vi "HostMain.vi"() -> ()   [LabVIEW 2017]
doc: "Main VI to be run from host computer. Can be started before or after the cRIO VI, RTMain.vi"
uses:
  RTControl/StateList.ctl
  HostDataGLOBAL.vi
  SystemsCheckPressureLimitGLOBAL.vi
  HostCurrentTimeGLOBAL.vi
  <vilib>/Utility/file.llb/Write Delimited Spreadsheet (string).vi
  <vilib>/Utility/file.llb/Write Delimited Spreadsheet (DBL).vi
panel:
  in  "Vent Tubing":bool
  out "Distance":dbl(slide) scale=0.0..1609.0
  in  "Skip System Check":bool
  in  "Stop System Check":bool
  in  "Enable Pod Power":string
  in  "Vent Tanks":bool
  out "Acceleration Graph":cluster{dbl[], dbl[]}(graph)
  out "Speed Graph":cluster{dbl[], dbl[]}(graph)
  out "Emergency Source":string
  out "Health Check 2":T1(array[cluster])=[{"String"="Distance (m)", "Numeric"=0.0, "Boolean"=FALSE}, {"String"="Piezo (V)", "Numeric"=0.0, "Boolean"=FALSE}, {"String"="Battery Voltage (V)", "Numeric"=0.0, "Boolean"=FALSE}, {"String"="Battery Current (I)", "Numeric"=0.0, "Boolean"=FALSE}, {"String"="Battery Power (W)", "Numeric"=0.0, "Boolean"=FALSE}, {"String"="Battery Temperature (C)", "Numeric"=0.0, "Boolean"=FALSE}, {"String"="cRIO Temperature (C)", "Numeric"=0.0, "Boolean"=FALSE}, {"String"="Right Big Tank Temperature (C)", "Numeric"=0.0, "Boolean"=FALSE}, {"String"="Left Big Tank Temperature (C)", "Numeric"=0.0, "Boolean"=FALSE}, {"String"="Baby Tank Temperature (C)", "Numeric"=0.0, "Boolean"=FALSE}, {"String"="Right Manifold Temperature (C)", "Numeric"=0.0, "Boolean"=FALSE}, {"String"="Left Manifold Temperature (C)", "Numeric"=0.0, "Boolean"=FALSE}, {"String"="IMU Acceleration", "Numeric"=0.0, "Boolean"=FALSE}, {"String"="IMU Pressure", "Numeric"=0.0, "Boolean"=FALSE}, {"String"="IMU Temperature", "Numeric"=0.0, "Boolean"=FALSE}]
  out "End Coast Time":dbl=-0.01
  out "End Push Time":dbl=-0.01
  out "Start Push Time":dbl=-0.01
  out "Current Time":dbl=-0.01
  in  "Force Idle":bool
  in  "Testing Mode?":bool
  out "Health Check":T1(array[cluster])=[{"String"="Suspension Pressure (PSI)", "Numeric"=0.0, "Boolean"=FALSE}, {"String"="MagBrake Pressure (PSI)", "Numeric"=0.0, "Boolean"=FALSE}, {"String"="Small Tank (PSI)", "Numeric"=0.0, "Boolean"=FALSE}, {"String"="Big Tank Right (PSI)", "Numeric"=0.0, "Boolean"=FALSE}, {"String"="Big Tank Left (PSI)", "Numeric"=0.0, "Boolean"=FALSE}, {"String"="FL Hall Effect (V)", "Numeric"=0.0, "Boolean"=FALSE}, {"String"="FR Hall Effect (V)", "Numeric"=0.0, "Boolean"=FALSE}, {"String"="BR Hall Effect (V)", "Numeric"=0.0, "Boolean"=FALSE}, {"String"="BL Hall Effect (V)", "Numeric"=0.0, "Boolean"=FALSE}, {"String"="FR Linear Pot (V)", "Numeric"=0.0, "Boolean"=FALSE}, {"String"="FL Linear Pot (V)", "Numeric"=0.0, "Boolean"=FALSE}, {"String"="BR Linear Pot (V)", "Numeric"=0.0, "Boolean"=FALSE}, {"String"="BL Linear Pot (V)", "Numeric"=0.0, "Boolean"=FALSE}, {"String"="Speed (m/s)", "Numeric"=0.0, "Boolean"=FALSE}]
  out "UDP String":string
  in  "Emergency":bool
  in  "Clear Error":bool
  in  "Abort":bool
  out "CurrentState":T2
  in  "Idle to Ready":bool
  in  "Power On":bool
  in  "Stop Host":bool
  in  "Stop cRIO":bool
  out "Solenoid Tabs":enum32{"System Check", "State Machine"}(tab)
  in  "All Toggle On":bool
  in  "All Toggle Off":bool
  in  "Manual Control":bool
  in  "NC09":bool
  in  "NO01":bool
  in  "NC08":bool
  in  "NC05":bool
  in  "NC06":bool
  in  "NC07":bool
  in  "NC03":bool
  in  "NC04":bool
  in  "NC02":bool
  in  "NC10":bool
  in  "NO02":bool
  in  "NC01":bool
  in  "Mag Brake Toggle":bool
  in  "Suspension Toggle":bool
  in  "Levitation Toggle":bool
  out "Left Solenoids":cluster{"String":string, "Boolean":bool}[](array[cluster])=[{"String"="NC03 FLSki", "Boolean"=FALSE}, {"String"="NC04 BLSki", "Boolean"=FALSE}, {"String"="NC02 BLSki", "Boolean"=FALSE}, {"String"="NC10 MagBr In", "Boolean"=FALSE}, {"String"="NO02 MagBr Out", "Boolean"=FALSE}, {"String"="NC01 FLSki", "Boolean"=FALSE}, {"String"="Pod Power", "Boolean"=FALSE}]
  out "Right Solenoids":cluster{"String":string, "Boolean":bool}[](array[cluster])=[{"String"="NC09 Susp In", "Boolean"=FALSE}, {"String"="NO01 Susp Out", "Boolean"=FALSE}, {"String"="NC08 BRSki", "Boolean"=FALSE}, {"String"="NC05 FRSki", "Boolean"=FALSE}, {"String"="NC06 BRSki", "Boolean"=FALSE}, {"String"="NC07 FRSki", "Boolean"=FALSE}, {"String"="NO03 All Out", "Boolean"=FALSE}, {"String"="Safety Panel", "Boolean"=FALSE}]
  # "IN"
  # "IN"
  # "MAG"
  # "SUSP"
  # "OUT"
  # "OUT"
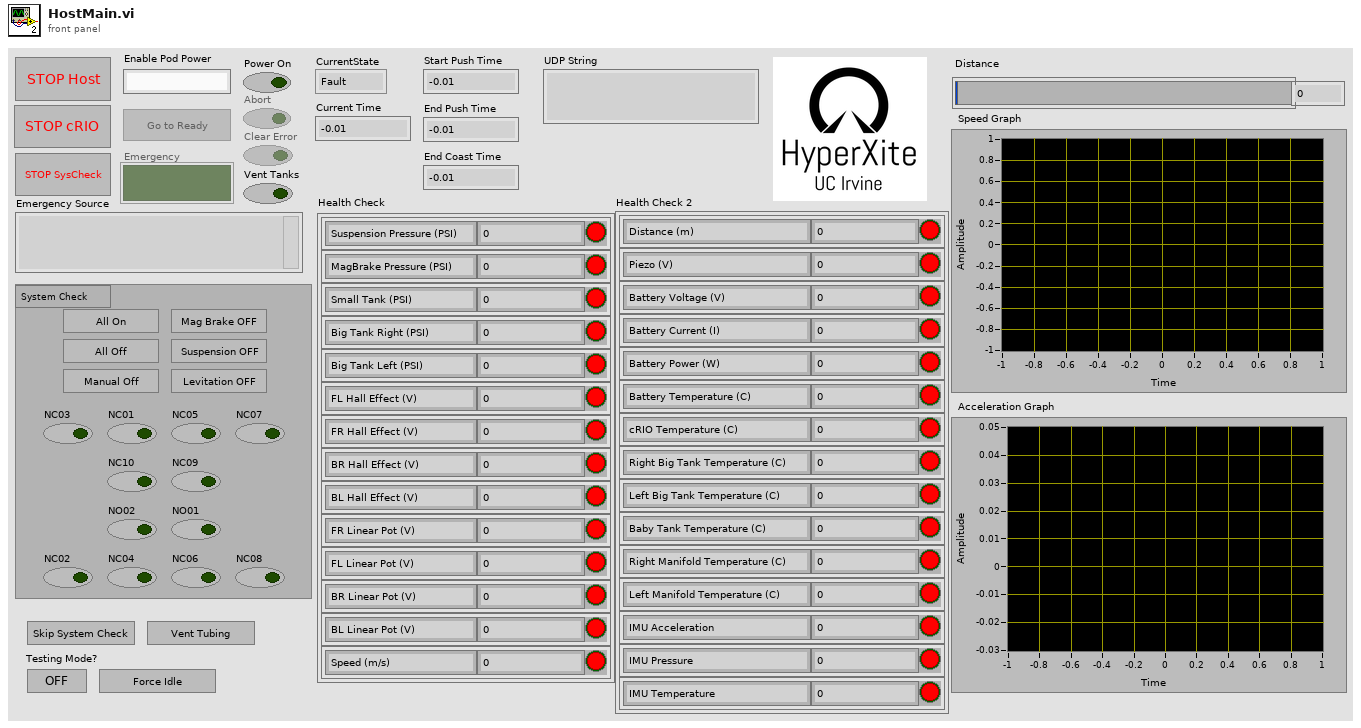
[diagram p1: front panel]
types:
  T1 = cluster{"String":string, "Numeric":dbl, "Boolean":bool}[]
  T2 = typedef "StateList.ctl" = enum16{"Fault", "Idle", "Ready", "Pushing", "Coast", "Braking"}
  T3 = enum8{"Enabled", "Disabled", "Disabled and Grayed Out"}
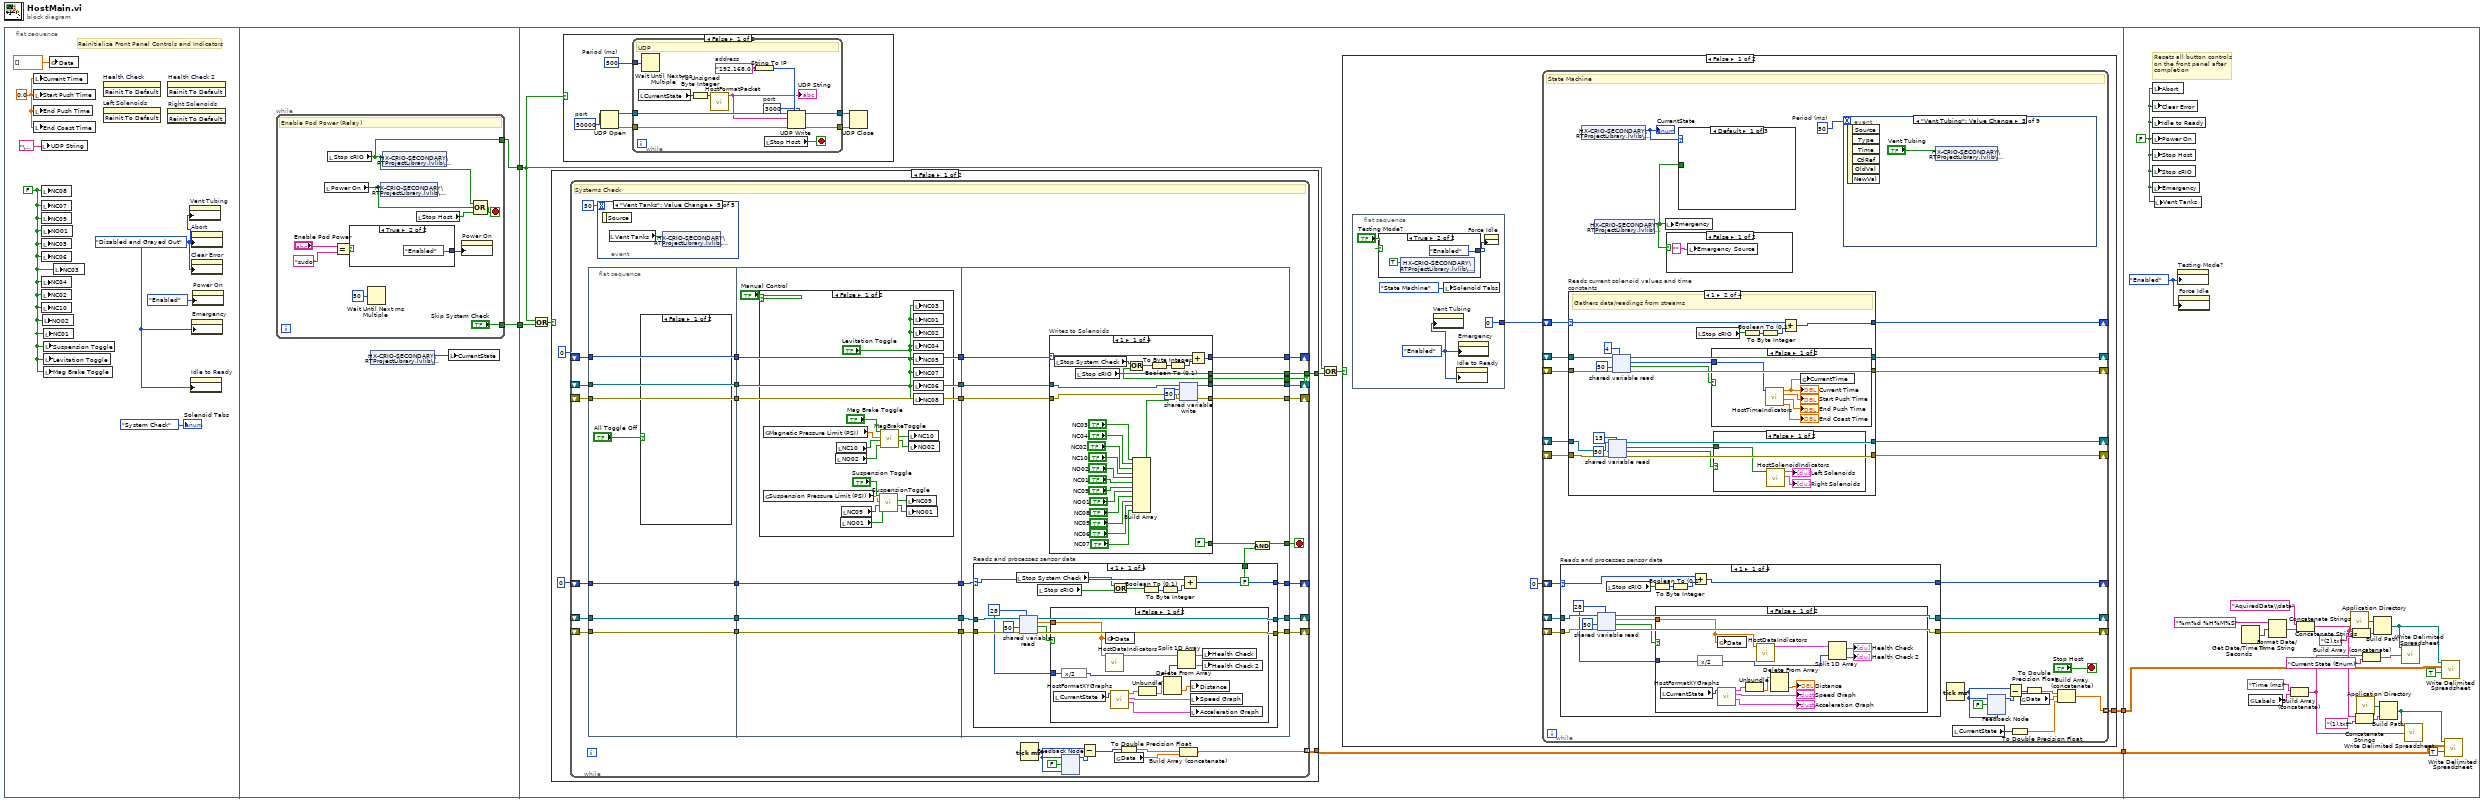
[diagram p0: block diagram]
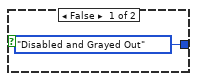
[diagram p2: hidden frame]
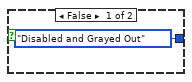
[diagram p4: hidden frame]
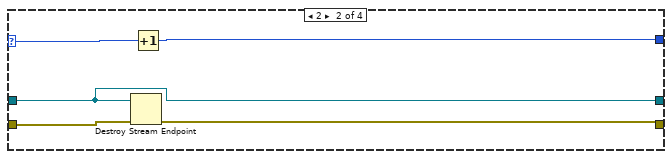
[diagram p6: hidden frame]
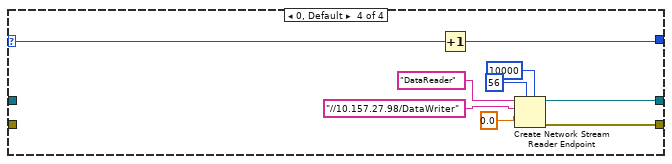
[diagram p8: hidden frame]
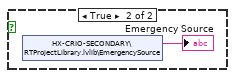
[diagram p9: hidden frame]
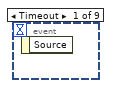
[diagram p10: hidden frame]
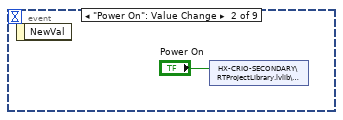
[diagram p11: hidden frame]
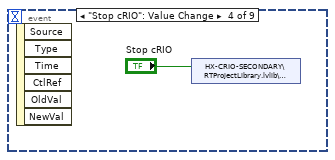
[diagram p12: hidden frame]
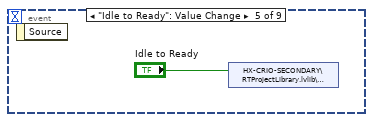
[diagram p13: hidden frame]
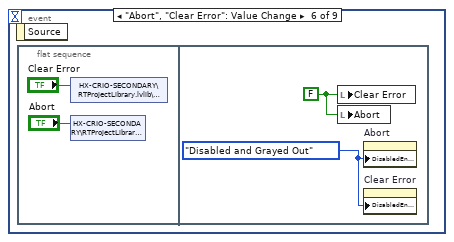
[diagram p14: hidden frame]
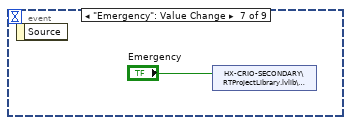
[diagram p15: hidden frame]
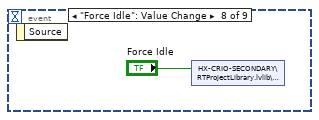
[diagram p16: hidden frame]
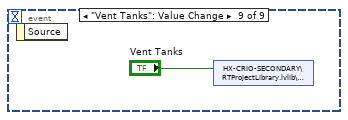
[diagram p17: hidden frame]
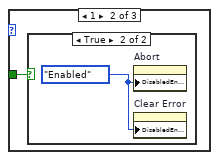
[diagram p18: hidden frame]
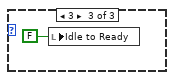
[diagram p20: hidden frame]
diagram:
  n1 = flat-sequence {
    tunnel: [w14] -> w4
    tunnel: [w13] -> w3
    tunnel: w4 -> [w32]
    tunnel: w3 -> [w27]
    tunnel: [w29] -> w2
    tunnel: [w28] -> w1
    tunnel: w2 -> [w412]
    tunnel: w1 -> [w411]
    frame #0 {
      w5 = T3."Disabled and Grayed Out" ("Disabled")
      w6 = FALSE
      w10 = 0.0 ("Speed (m/s)")
      # "Reinitialize Front Panel Controls and Indicators"
      n2 = local write "Current Time"(w10) -> ()
      n3 = local write "Start Push Time"(w10) -> ()
      n4 = local write "End Push Time"(w10) -> ()
      n5 = local write "End Coast Time"(w10) -> ()
      n6 = local write "UDP String"("\u0000\u0000\u0000\u0000\u0000\u0000\u0000\u0000\u0000\u0000\u0000\u0000\u0000\u0000\u0000\u0000\u0000\u0000\u0000\u0000\u0000\u0000\u0000\u0000\u0000\u0000\u0000\u0000\u0000\u0000\u0000\u0000\u0000\u0000" ("UDP String")) -> ()
      n7 = local write "NC08"(w6) -> ()
      n8 = local write "NC07"(w6) -> ()
      n9 = local write "NC09"(w6) -> ()
      n10 = local write "NO01"(w6) -> ()
      n11 = local write "NC05"(w6) -> ()
      n12 = local write "NC06"(w6) -> ()
      n13 = local write "NC04"(w6) -> ()
      n14 = local write "NC02"(w6) -> ()
      n15 = local write "NC10"(w6) -> ()
      n16 = local write "NO02"(w6) -> ()
      n17 = local write "NC01"(w6) -> ()
      n18 = local write "Suspension Toggle"(w6) -> ()
      n19 = local write "Levitation Toggle"(w6) -> ()
      n20 = local write "Mag Brake Toggle"(w6) -> ()
      n21 = global write "HostDataGLOBAL.vi" "Data"(dbl[] [] ("Data")) -> ()
      n22 = local write "NC03"(w6) -> ()
      n23 = invoke on="Health Check" class="Arr (strict)" method="Reinit To Default"() -> ()  [unwired: 3 in, 3 out]
      n24 = invoke on="Left Solenoids" class="Arr (strict)" method="Reinit To Default"() -> ()  [unwired: 3 in, 3 out]
      n25 = invoke on="Health Check 2" class="Arr (strict)" method="Reinit To Default"() -> ()  [unwired: 3 in, 3 out]
      n26 = invoke on="Right Solenoids" class="Arr (strict)" method="Reinit To Default"() -> ()  [unwired: 3 in, 3 out]
      n27 = property on="Vent Tubing" class="Bool (strict)"("DisabledEnum"=w5) -> ()  [unwired: 2 in, 2 out]
      n28 = property on="Idle to Ready" class="Bool (strict)"("DisabledEnum"=w5) -> ()  [unwired: 2 in, 2 out]
      n29 = property on="Abort" class="Bool (strict)"("DisabledEnum"=w5) -> ()  [unwired: 2 in, 2 out]
      n30 = property on="Clear Error" class="Bool (strict)"("DisabledEnum"=w5) -> ()  [unwired: 2 in, 2 out]
      n31 = property on="Emergency" class="Bool (strict)"("DisabledEnum"=w5) -> ()  [unwired: 2 in, 2 out]
      n32 = property on="Power On" class="Bool (strict)"("DisabledEnum"=T3."Enabled" ("Disabled")) -> ()  [unwired: 2 in, 2 out]
      "Solenoid Tabs" <- enum32{"System Check", "State Machine"}."System Check" ("Solenoid Tabs")
    }
    frame #1 {
      n33 = while {
        tunnel: ["Skip System Check"] -> w14
        tunnel: [w15] -> w13
        stop <- w23 stop-if-true
        # "Enable Pod Power (Relay)"
        n34 = local read "Power On"() -> (w16:bool)
        n35 = local read "Stop cRIO"() -> (w15:bool)
        n36 = Equal?(x="Enable Pod Power", y="sudo") -> (x = y?=w19:bool)
        n37 = case shown="True" w19 {
          tunnel: [T3."Disabled and Grayed Out" ("Disabled") T3."Enabled" ("Disabled")] -> w18
          frame False {
          }
          frame True {
          }
        }
        n38 = Wait Until Next ms Multiple(millisecond multiple=u32 50) -> ()  [unwired: 1 out]
        n39 = shared-variable "HX-CRIO-SECONDARY\\RTProjectLibrary.lvlib\\PodPower"(w16) -> ()  [unwired: 1 in, 1 out]
        n40 = shared-variable "HX-CRIO-SECONDARY\\RTProjectLibrary.lvlib\\StopControl"(w15) -> ()  [unwired: 1 in, 1 out]
        n41 = local read "Stop Host"() -> (w24:bool)
        n42 = property on="Power On" class="Bool (strict)"("DisabledEnum"=w18) -> ()  [unwired: 2 in, 2 out]
        n43 = Compound Arithmetic op=OR(w15, w16, w24) -> (w23:bool)
      }
      n44 = shared-variable "HX-CRIO-SECONDARY\\RTProjectLibrary.lvlib\\CurrentState"() -> (w12:u8)  [unwired: 1 in, 1 out]
      n45 = local write "CurrentState"(w12) -> ()
    }
    frame #2 {
      n46 = Or(x=w27, y=w32) -> (x .or. y?=w33:bool)
      n47 = case shown="False" w33 {
        selector: w33 -> [_ w399]
        tunnel: [w211 FALSE ("Stop cRIO")] -> w31
        tunnel: [w210 dbl[][] [] ("Data")] -> w28
        frame False {
          n48 = while {
            shift-right: [w246] -> _
            shift-left: i8 0 -> [w247]
            shift-right: [w245] -> _
            shift-left: _ -> [w243]
            shift-right: [w244] -> _
            shift-left: _ -> [w242]
            tunnel: [w233] -> w211 if=w232
            shift-right: [w228] -> _
            shift-left: i8 0 -> [w229]
            shift-right: [w221] -> _
            shift-left: _ -> [w225]
            shift-right: [w220] -> _
            shift-left: _ -> [w222]
            tunnel: [w218] -> w210 mode=indexing
            stop <- w241 stop-if-true
            # "Systems Check"
            n49 = flat-sequence {
              tunnel: w242 -> [w256]
              tunnel: w243 -> [w257]
              tunnel: w247 -> [w258]
              tunnel: [w258] -> w237
              tunnel: [w257] -> w236
              tunnel: [w256] -> w235
              tunnel: [w254] -> w230
              tunnel: w229 -> [w254]
              tunnel: [w253] -> w226
              tunnel: w225 -> [w253]
              tunnel: [w252] -> w223
              tunnel: w222 -> [w252]
              tunnel: [w267] -> w240
              tunnel: [w266] -> w239
              tunnel: [w265] -> w238
              tunnel: w237 -> [w267]
              tunnel: w236 -> [w266]
              tunnel: w235 -> [w265]
              tunnel: [w263] -> w231
              tunnel: w230 -> [w263]
              tunnel: [w262] -> w227
              tunnel: w226 -> [w262]
              tunnel: [w261] -> w224
              tunnel: w223 -> [w261]
              tunnel: [w298] -> w246
              tunnel: [w297] -> w245
              tunnel: [w296] -> w244
              tunnel: [w284] -> w241
              tunnel: w240 -> [w299]
              tunnel: w239 -> [w295]
              tunnel: w238 -> [w294]
              tunnel: [w292] -> w233
              tunnel: [w291] -> w232
              tunnel: w231 -> [w290]
              tunnel: [w289] -> w228
              tunnel: w227 -> [w288]
              tunnel: w224 -> [w287]
              tunnel: [w286] -> w221
              tunnel: [w285] -> w220
              frame #0 {
                n50 = case shown="False" "All Toggle Off" {
                  selector: "All Toggle Off" -> [_ w260]
                  frame False {
                  }
                  frame True {
                    n51 = Not(x=w260) -> (.not. x?=w259:bool)
                    n52 = local write "Suspension Toggle"(w259) -> ()
                    n53 = local write "Mag Brake Toggle"(w259) -> ()
                    n54 = local write "Levitation Toggle"(w259) -> ()
                    n55 = local write "NO01"(w259) -> ()
                    n56 = local write "NO02"(w259) -> ()
                    n57 = local write "NC08"(w259) -> ()
                    n58 = local write "NC07"(w259) -> ()
                    n59 = local write "NC09"(w259) -> ()
                    n60 = local write "NC05"(w259) -> ()
                    n61 = local write "NC06"(w259) -> ()
                    n62 = local write "NC03"(w259) -> ()
                    n63 = local write "NC04"(w259) -> ()
                    n64 = local write "NC02"(w259) -> ()
                    n65 = local write "NC10"(w259) -> ()
                    n66 = local write "NC01"(w259) -> ()
                  }
                }
              }
              frame #1 {
                n67 = case shown="False" "Manual Control" {
                  frame False {
                    n68 = global read "SystemsCheckPressureLimitGLOBAL.vi" "Magnetic Pressure Limit (PSI)"() -> (w269:dbl)
                    n69 = global read "SystemsCheckPressureLimitGLOBAL.vi" "Suspension Pressure Limit (PSI)"() -> (w268:dbl)
                    n70 = local read "NO02"() -> (w278:bool)
                    n71 = local read "NC10"() -> (w277:bool)
                    n72 = local read "NO01"() -> (w280:bool)
                    n73 = local read "NC09"() -> (w279:bool)
                    n74 = call "SuspensionToggle.vi"("Susp Out"=w280, "SuspIn"=w279, "Suspension Pressure Limit (PSI)"=w268, "SuspensionOn?"="Suspension Toggle") -> ("SuspOut"=w275:bool, "SuspIn"=w276:bool)  [unwired: 5 in, 1 out]
                    n75 = call "MagBrakeToggle.vi"("MagBrake Out"=w278, "MagBrake In"=w277, "MagPressureLimit (PSI)"=w269, "MagBrakeOn?"="Mag Brake Toggle") -> ("MagBrake OUTPUT"=w274:bool, "MagBrake In"=w273:bool)  [unwired: 5 in, 1 out]
                    n76 = local write "NC09"(w276) -> ()
                    n77 = local write "NO01"(w275) -> ()
                    n78 = local write "NC10"(w273) -> ()
                    n79 = local write "NO02"(w274) -> ()
                    n80 = local write "NC03"("Levitation Toggle") -> ()
                    n81 = local write "NC01"("Levitation Toggle") -> ()
                    n82 = local write "NC02"("Levitation Toggle") -> ()
                    n83 = local write "NC04"("Levitation Toggle") -> ()
                    n84 = local write "NC05"("Levitation Toggle") -> ()
                    n85 = local write "NC07"("Levitation Toggle") -> ()
                    n86 = local write "NC06"("Levitation Toggle") -> ()
                    n87 = local write "NC08"("Levitation Toggle") -> ()
                  }
                  frame True {
                    n88 = case shown="True" "All Toggle On" {
                      selector: "All Toggle On" -> [_ w282]
                      frame False {
                      }
                      frame True {
                        n89 = local write "NC08"(w282) -> ()
                        n90 = local write "NC07"(w282) -> ()
                        n91 = local write "NC09"(w282) -> ()
                        n92 = local write "NO01"(w282) -> ()
                        n93 = local write "NC05"(w282) -> ()
                        n94 = local write "NC06"(w282) -> ()
                        n95 = local write "NC03"(w282) -> ()
                        n96 = local write "NC04"(w282) -> ()
                        n97 = local write "NC02"(w282) -> ()
                        n98 = local write "NC10"(w282) -> ()
                        n99 = local write "NO02"(w282) -> ()
                        n100 = local write "NC01"(w282) -> ()
                      }
                    }
                  }
                }
              }
              frame #2 {
                n101 = case "Reads and processes sensor data" shown="1" w290 {
                  selector: w290 -> [w310 w333 w337 w343]
                  tunnel: [w311 w332 w337 w342] -> w289
                  tunnel: [w309 w329 w336 w341] -> w286
                  tunnel: [w308 w330 w335 w340] -> w285
                  tunnel: w288 -> [w312 w329 w336 _]
                  tunnel: w287 -> [w313 w331 w335 _]
                  tunnel: [FALSE FALSE TRUE FALSE] -> w283
                  frame 1 {
                    w303 = 28 ("# elements")
                    n102 = local read "Stop System Check"() -> (w304:bool)
                    n103 = shared-variable-read(w312, w313, 50 ("timeout ms (-1)"), w303) -> (w309:refnum<k21>, w308:errorcluster, w300:bool, w302:dbl[])
                    n104 = local read "Stop cRIO"() -> (w306:bool)
                    n105 = case shown="False" w300 {
                      tunnel: w303 -> [w323 _]
                      tunnel: w302 -> [w321 _]
                      frame False {
                        n106 = local read "CurrentState"() -> (w325:T2)
                        n107 = expression code="x/2"(w323) -> (w324:i32)
                        n108 = global write "HostDataGLOBAL.vi" "Data"(w321) -> ()
                        n109 = call "HostDataIndicators.vi"("Array"=w321) -> ("Health Check"=w322:T1)  [unwired: 10 in]
                        n110 = call "HostFormatXYGraphs.vi"("CurrentState"=w325) -> ("Acceleration Graph"=w318:cluster{dbl[], dbl[]}, "Speed Graph"=w317:cluster{dbl[], dbl[]}, "Distance Graph"=w326:cluster{dbl[], dbl[]})  [unwired: 8 in]
                        n111 = Unbundle(w326) -> (w327:dbl[])  [unwired: 1 out]
                        n112 = Delete From Array(array=w327) -> (deleted portion=w316:dbl)  [unwired: 2 in, 1 out]
                        n113 = Split 1D Array(array=w322, index=w324) -> (first subarray=w320:T1, second subarray=w319:T1)
                        n114 = local write "Distance"(w316) -> ()
                        n115 = local write "Speed Graph"(w317) -> ()
                        n116 = local write "Acceleration Graph"(w318) -> ()
                        n117 = local write "Health Check"(w320) -> ()
                        n118 = local write "Health Check 2"(w319) -> ()
                      }
                      frame True {
                      }
                    }
                    n119 = Or(x=w304, y=w306) -> (x .or. y?=w305:bool)
                    n120 = Boolean To (0,1)(Boolean=w305) -> (0, 1=w314:i16)
                    n121 = To Byte Integer(number=w314) -> (8bit integer=w315:i8)
                    n122 = Add(x=w310, y=w315) -> (x+y=w311:i8)
                  }
                  frame 2 {
                    n123 = Destroy Stream Endpoint(8:w331, 11:w329) -> (0:w330:errorcluster)
                    n124 = Increment(x=w333) -> (x+1=w332:i8)
                  }
                  frame 3 {
                  }
                  frame 0, Default {
                    n125 = Increment(x=w343) -> (x+1=w342:i8)
                    n126 = Create Network Stream Reader Endpoint(5:10000 ("timeout in ms (-1)"), 7:56 ("reader buffer size"), 9:0.0, 10:"//10.157.27.98/DataWriter" ("writer url"), 11:"DataReader" ("reader name")) -> (0:w340:errorcluster, 3:w341:refnum<k21>)  [unwired: 2 in]
                  }
                }
                n127 = case "Writes to Solenoids" shown="1" w299 {
                  selector: w299 -> [w371 w377 w381 w392]
                  tunnel: [w368 w374 w381 w391] -> w298
                  tunnel: [w369 w378 w383 w390] -> w297
                  tunnel: [w370 w379 w384 w389] -> w296
                  tunnel: w295 -> [w349 w378 w383 _]
                  tunnel: w294 -> [w350 w380 w384 _]
                  tunnel: [FALSE FALSE TRUE FALSE] -> w293
                  tunnel: [w353 w375 w382 FALSE ("Stop cRIO")] -> w292
                  tunnel: [w353 w375 w382 TRUE ("Stop cRIO")] -> w291
                  frame 1 {
                    n128 = local read "Stop System Check"() -> (w351:bool)
                    n129 = local read "Stop cRIO"() -> (w353:bool)
                    n130 = Or(x=w351, y=w353) -> (x .or. y?=w352:bool)
                    n131 = Build Array("NC03", "NC04", "NC02", "NC10", "NO02", "NC01", "NC09", "NO01", "NC08", "NC05", "NC06", "NC07") -> (w355:bool[])
                    n132 = Boolean To (0,1)(Boolean=w352) -> (0, 1=w372:i16)
                    n133 = To Byte Integer(number=w372) -> (8bit integer=w373:i8)
                    n134 = shared-variable-write(w349, w350, w355, 50 ("timeout ms (-1)")) -> (w369:refnum<k21>, w370:errorcluster)  [unwired: 1 out]
                    n135 = Add(x=w371, y=w373) -> (x+y=w368:i8)
                  }
                  frame 2 {
                    w375 = FALSE ("Stop cRIO")
                    n136 = Destroy Stream Endpoint(8:w380, 11:w378) -> (0:w379:errorcluster)
                    n137 = Increment(x=w377) -> (x+1=w374:i8)
                  }
                  frame 3 {
                    w382 = FALSE ("Stop cRIO")
                  }
                  frame 0, Default {
                    n138 = Increment(x=w392) -> (x+1=w391:i8)
                    n139 = Create Network Stream Writer Endpoint(7:24 ("reader buffer size"), 9:FALSE, 10:"//10.157.27.98/ManuelWriter" ("writer url"), 11:"ManuelReader" ("reader name")) -> (0:w389:errorcluster, 3:w390:refnum<k21>)  [unwired: 3 in]
                  }
                }
                n140 = And(x=w293, y=w283) -> (x .and. y?=w284:bool)
              }
            }
            n141 = event shown="[4] \"Vent Tanks\": Value Change" {
              selector: _ -> [_ _ _ _ _]
              dyn-events: _ -> [_ _ _ _ _]
              timeout: 50 -> [_ _ _ _ _]
              event Timeout {
                n142 = event-data() -> ()  [unwired: 1 in, 1 out]
              }
              event "Stop System Check": Value Change {
                n143 = event-data() -> ()  [unwired: 1 in, 1 out]
                n144 = shared-variable "HX-CRIO-SECONDARY\\RTProjectLibrary.lvlib\\StopSystemCheck"("Stop System Check") -> ()  [unwired: 1 in, 1 out]
              }
              event "Power On": Value Change {
                n145 = event-data() -> ()  [unwired: 1 in, 1 out]
                n146 = local read "Power On"() -> (w249:bool)
                n147 = shared-variable "HX-CRIO-SECONDARY\\RTProjectLibrary.lvlib\\PodPower"(w249) -> ()  [unwired: 1 in, 1 out]
              }
              event "Stop cRIO": Value Change {
                n148 = event-data() -> ()  [unwired: 1 in, 1 out]
                n149 = local read "Stop cRIO"() -> (w250:bool)
                n150 = shared-variable "HX-CRIO-SECONDARY\\RTProjectLibrary.lvlib\\StopControl"(w250) -> ()  [unwired: 1 in, 1 out]
              }
              event "Vent Tanks": Value Change {
                n151 = event-data() -> ()  [unwired: 1 in, 1 out]
                n152 = local read "Vent Tanks"() -> (w251:bool)
                n153 = shared-variable "HX-CRIO-SECONDARY\\RTProjectLibrary.lvlib\\VentTanks"(w251) -> ()  [unwired: 1 in, 1 out]
              }
            }
            n154 = Tick Count (ms)() -> (millisecond timer value=w214:u32)
            n155 = feedback-in #1(w214, FALSE) -> ()
            n156 = feedback #1(w214) -> (w217:u32)
            n157 = Subtract(x=w214, y=w217) -> (x-y=w216:u32)
            n158 = global read "HostDataGLOBAL.vi" "Data"() -> (w219:dbl[])
            n159 = To Double Precision Float(number=w216) -> (double precision float=w215:dbl)
            n160 = Build Array (concatenate)(w215, w219) -> (w218:dbl[])
          }
        }
        frame True {
          n161 = shared-variable "HX-CRIO-SECONDARY\\RTProjectLibrary.lvlib\\StopSystemCheck"(w399) -> ()  [unwired: 1 in, 1 out]
        }
      }
      n162 = case shown="False" w27 {
        frame False {
          w34 = u32 500  # Period (ms)
          w35 = u16 50000  # port
          n163 = UDP Open(11:w35) -> (port=w36:refnum<k16>, 0:w39:errorcluster)  [unwired: 4 in, 1 out]
          n164 = while {
            tunnel: w39 -> [w50]
            tunnel: [w49] -> w38
            tunnel: [w48] -> w37
            tunnel: w36 -> [w47]
            tunnel: w34 -> [w40]
            stop <- w51 stop-if-true
            w44 = u16 3000  # port
            w45 = "192.168.0.1"  # address
            # "UDP"
            n165 = local read "CurrentState"() -> (w42:T2)
            n166 = Wait Until Next ms Multiple(millisecond multiple=w40) -> ()  [unwired: 1 out]
            n167 = To Unsigned Byte Integer(number=w42) -> (unsigned 8bit integer=w41:u8)
            n168 = call "HostFormatPacket.vi"("Enum in"=w41) -> ("data string"=w43:string)  [unwired: 10 in]
            "UDP String" <- w43
            n169 = String To IP(1:w45) -> (0:w46:u32)
            n170 = local read "Stop Host"() -> (w51:bool)
            n171 = UDP Write(address=w46, port or service name=w44, connection ID=w47, data in=w43, 8:w50) -> (error out=w49:errorcluster, 3:w48:refnum<k16>)  [unwired: 1 in]
          }
          n172 = UDP Close(connection ID=w37, 8:w38) -> ()  [unwired: 2 out]
        }
        frame True {
        }
      }
      n173 = Or(x=w27, y=w31) -> (x .or. y?=w30:bool)
      n174 = case shown="False" w30 {
        tunnel: [w53 dbl[][] [] ("Data")] -> w29
        frame False {
          n175 = flat-sequence {
            tunnel: [i8 0] -> w54
            frame #0 {
              w55 = T3."Enabled" ("Disabled")
              n176 = case shown="True" "Testing Mode?" {
                tunnel: [T3."Disabled and Grayed Out" ("Disabled") T3."Enabled" ("Disabled")] -> w58
                frame False {
                }
                frame True {
                  n177 = shared-variable "HX-CRIO-SECONDARY\\RTProjectLibrary.lvlib\\EnableForceIdle"(TRUE ("EnableForceIdle")) -> ()  [unwired: 1 in, 1 out]
                }
              }
              n178 = property on="Vent Tubing" class="Bool (strict)"("DisabledEnum"=w55) -> ()  [unwired: 2 in, 2 out]
              n179 = local write "Solenoid Tabs"(enum32{"System Check", "State Machine"}."State Machine" ("Solenoid Tabs")) -> ()
              n180 = property on="Idle to Ready" class="Bool (strict)"("DisabledEnum"=w55) -> ()  [unwired: 2 in, 2 out]
              n181 = property on="Emergency" class="Bool (strict)"("DisabledEnum"=w55) -> ()  [unwired: 2 in, 2 out]
              n182 = property on="Force Idle" class="Bool"("DisabledEnum"=w58) -> ()  [unwired: 2 in, 2 out]
            }
          }
          n183 = while {
            shift-right: [w90] -> _
            shift-left: _ -> [w88]
            shift-right: [w89] -> _
            shift-left: _ -> [w87]
            shift-right: [w83] -> _
            shift-left: w54 -> [w86]
            shift-right: [w80] -> _
            shift-left: _ -> [w82]
            shift-right: [w79] -> _
            shift-left: _ -> [w81]
            shift-right: [w74] -> _
            shift-left: i8 0 -> [w77]
            shift-right: [w73] -> _
            shift-left: _ -> [w76]
            shift-right: [w72] -> _
            shift-left: _ -> [w75]
            tunnel: [w65] -> w53 mode=indexing
            stop <- "Stop Host" stop-if-true
            w84 = 50  # Period (ms)
            # "State Machine"
            n184 = case "Reads and processes sensor data" shown="1" w77 {
              selector: w77 -> [w98 w121 w124 w129]
              tunnel: [w99 w120 w124 w128] -> w74
              tunnel: [w97 w117 w123 w127] -> w73
              tunnel: [w96 w118 w122 w126] -> w72
              tunnel: w76 -> [w100 w117 w123 _]
              tunnel: w75 -> [w101 w119 w122 _]
              frame 1 {
                w95 = 28 ("# elements")
                n185 = shared-variable-read(w100, w101, 50 ("timeout ms (-1)"), w95) -> (w97:refnum<k21>, w96:errorcluster, w92:bool, w94:dbl[])
                n186 = local read "Stop cRIO"() -> (w104:bool)
                n187 = Boolean To (0,1)(Boolean=w104) -> (0, 1=w102:i16)
                n188 = case shown="False" w92 {
                  tunnel: w95 -> [w112 _]
                  tunnel: w94 -> [w110 _]
                  frame False {
                    n189 = local read "CurrentState"() -> (w114:T2)
                    n190 = expression code="x/2"(w112) -> (w113:i32)
                    n191 = call "HostFormatXYGraphs.vi"("CurrentState"=w114) -> ("Acceleration Graph"=→"Acceleration Graph":cluster{dbl[], dbl[]}, "Speed Graph"=→"Speed Graph":cluster{dbl[], dbl[]}, "Distance Graph"=w115:cluster{dbl[], dbl[]})  [unwired: 8 in]
                    n192 = global write "HostDataGLOBAL.vi" "Data"(w110) -> ()
                    n193 = Unbundle(w115) -> (w116:dbl[])  [unwired: 1 out]
                    n194 = call "HostDataIndicators.vi"("Array"=w110) -> ("Health Check"=w111:T1)  [unwired: 10 in]
                    n195 = Delete From Array(array=w116) -> (deleted portion=→"Distance":dbl)  [unwired: 2 in, 1 out]
                    n196 = Split 1D Array(array=w111, index=w113) -> (first subarray=→"Health Check":T1, second subarray=→"Health Check 2":T1)
                  }
                  frame True {
                  }
                }
                n197 = To Byte Integer(number=w102) -> (8bit integer=w103:i8)
                n198 = Add(x=w98, y=w103) -> (x+y=w99:i8)
              }
              frame 2 {
                n199 = Destroy Stream Endpoint(8:w119, 11:w117) -> (0:w118:errorcluster)
                n200 = Increment(x=w121) -> (x+1=w120:i8)
              }
              frame 3 {
              }
              frame 0, Default {
                n201 = Increment(x=w129) -> (x+1=w128:i8)
                n202 = Create Network Stream Reader Endpoint(5:10000 ("timeout in ms (-1)"), 7:56 ("reader buffer size"), 9:0.0, 10:"//10.157.27.98/DataWriter" ("writer url"), 11:"DataReader" ("reader name")) -> (0:w126:errorcluster, 3:w127:refnum<k21>)  [unwired: 2 in]
              }
            }
            n203 = case "Reads current solenoid values and time constants" shown="1" w86 {
              selector: w86 -> [w153 w178 w202 w207]
              tunnel: [w161 w186 w199 w205] -> w90
              tunnel: [w160 w185 w201 w206] -> w89
              tunnel: w87 -> [_ w175 w200 w206]
              tunnel: w88 -> [_ w174 w199 w205]
              tunnel: [w152 w177 w195 w207] -> w83
              tunnel: w82 -> [_ w184 w196 w204]
              tunnel: w81 -> [_ w176 w197 w203]
              tunnel: [w155 w183 w196 w204] -> w80
              tunnel: [w154 w182 w198 w203] -> w79
              frame 0, Default {
                # "Initializes streams"
                n204 = Increment(x=w153) -> (x+1=w152:i8)
                n205 = Create Network Stream Reader Endpoint(5:10000 ("timeout in ms (-1)"), 7:8 ("reader buffer size"), 9:i64 0, 10:"//10.157.27.98/TimeWriter" ("writer url"), 11:"TimeReader" ("reader name")) -> (0:w154:errorcluster, 3:w155:refnum<k21>)  [unwired: 2 in]
                n206 = Create Network Stream Reader Endpoint(5:10000 ("timeout in ms (-1)"), 7:30 ("reader buffer size"), 9:FALSE, 10:"//10.157.27.98/ControlWriter" ("writer url"), 11:"ControlReader" ("reader name")) -> (0:w160:errorcluster, 3:w161:refnum<k21>)  [unwired: 2 in]
              }
              frame 1 {
                # "Gathers data/readings from streams"
                n207 = shared-variable-read(w174, w175, 50 ("timeout ms (-1)"), 15 ("# elements")) -> (w186:refnum<k21>, w185:errorcluster, w166:bool, w170:bool[])
                n208 = shared-variable-read(w184, w176, 50 ("timeout ms (-1)"), 4 ("# elements")) -> (w183:refnum<k21>, w182:errorcluster, w167:bool, w172:i64[])
                n209 = local read "Stop cRIO"() -> (w179:bool)
                n210 = case shown="False" w167 {
                  tunnel: w172 -> [w194 _]
                  frame False {
                    n211 = call "HostTimeIndicators.vi"("Array"=w194) -> ("End Coast Time"=→"End Coast Time":dbl, "End Push Time"=→"End Push Time":dbl, "Start Push Time"=→"Start Push Time":dbl, "Current Time"=w190:dbl)  [unwired: 7 in]
                    "Current Time" <- w190
                    n212 = global write "HostCurrentTimeGLOBAL.vi" "CurrentTime"(w190) -> ()
                  }
                  frame True {
                  }
                }
                n213 = case shown="False" w166 {
                  tunnel: w170 -> [w189 _]
                  frame False {
                    n214 = call "HostSolenoidIndicators.vi"("Array in"=w189) -> ("Right Solenoids"=→"Right Solenoids":cluster{string, bool}[], "Left Solenoids"=→"Left Solenoids":cluster{string, bool}[])  [unwired: 9 in]
                  }
                  frame True {
                  }
                }
                n215 = Boolean To (0,1)(Boolean=w179) -> (0, 1=w181:i16)
                n216 = To Byte Integer(number=w181) -> (8bit integer=w180:i8)
                n217 = Add(x=w178, y=w180) -> (x+y=w177:i8)
              }
              frame 2 {
                # "Terminates streams following pod shutdown command"
                n218 = Increment(x=w202) -> (x+1=w195:i8)
                n219 = Destroy Stream Endpoint(8:w197, 11:w196) -> (0:w198:errorcluster)
                n220 = Destroy Stream Endpoint(8:w200, 11:w199) -> (0:w201:errorcluster)
              }
              frame 3 {
                # "Waits until VI terminates"
              }
            }
            n221 = shared-variable "HX-CRIO-SECONDARY\\RTProjectLibrary.lvlib\\CurrentState"() -> (w85:u8)  [unwired: 1 in, 1 out]
            "CurrentState" <- w85
            n222 = shared-variable "HX-CRIO-SECONDARY\\RTProjectLibrary.lvlib\\Emergency"() -> (w78:bool)  [unwired: 1 in, 1 out]
            n223 = local write "Emergency"(w78) -> ()
            n224 = case shown="False" w78 {
              frame False {
                n225 = local write "Emergency Source"("" ("Emergency Source")) -> ()
              }
              frame True {
                n226 = shared-variable "HX-CRIO-SECONDARY\\RTProjectLibrary.lvlib\\EmergencySource"() -> (→"Emergency Source":string)  [unwired: 1 in, 1 out]
              }
            }
            n227 = case shown="Default" w85 {
              tunnel: w78 -> [_ w147 _]
              frame Default {
              }
              frame 1 {
                n228 = case shown="True" w147 {
                  frame False {
                  }
                  frame True {
                    w148 = T3."Enabled" ("Disabled")
                    n229 = property on="Abort" class="Bool (strict)"("DisabledEnum"=w148) -> ()  [unwired: 2 in, 2 out]
                    n230 = property on="Clear Error" class="Bool (strict)"("DisabledEnum"=w148) -> ()  [unwired: 2 in, 2 out]
                  }
                }
              }
              frame 3 {
                n231 = local write "Idle to Ready"(FALSE) -> ()
              }
            }
            n232 = event shown="[2] \"Vent Tubing\": Value Change" {
              selector: _ -> [_ _ _ _ _ _ _ _ _]
              dyn-events: _ -> [_ _ _ _ _ _ _ _ _]
              timeout: w84 -> [_ _ _ _ _ _ _ _ _]
              event Timeout {
                n233 = event-data() -> ()  [unwired: 1 in, 1 out]
              }
              event "Power On": Value Change {
                n234 = event-data() -> ()  [unwired: 1 in, 1 out]
                n235 = shared-variable "HX-CRIO-SECONDARY\\RTProjectLibrary.lvlib\\PodPower"("Power On") -> ()  [unwired: 1 in, 1 out]
              }
              event "Vent Tubing": Value Change {
                n236 = event-data() -> ()  [unwired: 1 in, 6 out]
                n237 = shared-variable "HX-CRIO-SECONDARY\\RTProjectLibrary.lvlib\\VentTubing"("Vent Tubing") -> ()  [unwired: 1 in, 1 out]
              }
              event "Stop cRIO": Value Change {
                n238 = event-data() -> ()  [unwired: 1 in, 6 out]
                n239 = shared-variable "HX-CRIO-SECONDARY\\RTProjectLibrary.lvlib\\StopControl"("Stop cRIO") -> ()  [unwired: 1 in, 1 out]
              }
              event "Idle to Ready": Value Change {
                n240 = event-data() -> ()  [unwired: 1 in, 1 out]
                n241 = shared-variable "HX-CRIO-SECONDARY\\RTProjectLibrary.lvlib\\IdleToReady"("Idle to Ready") -> ()  [unwired: 1 in, 1 out]
              }
              event "Abort", "Clear Error": Value Change {
                n242 = event-data() -> ()  [unwired: 1 in, 1 out]
                n243 = flat-sequence {
                  frame #0 {
                    n244 = shared-variable "HX-CRIO-SECONDARY\\RTProjectLibrary.lvlib\\ClearError"("Clear Error") -> ()  [unwired: 1 in, 1 out]
                    n245 = shared-variable "HX-CRIO-SECONDARY\\RTProjectLibrary.lvlib\\Abort"("Abort") -> ()  [unwired: 1 in, 1 out]
                  }
                  frame #1 {
                    w142 = T3."Disabled and Grayed Out" ("Disabled")
                    w143 = FALSE ("Abort")
                    n246 = local write "Clear Error"(w143) -> ()
                    n247 = local write "Abort"(w143) -> ()
                    n248 = property on="Abort" class="Bool (strict)"("DisabledEnum"=w142) -> ()  [unwired: 2 in, 2 out]
                    n249 = property on="Clear Error" class="Bool (strict)"("DisabledEnum"=w142) -> ()  [unwired: 2 in, 2 out]
                  }
                }
              }
              event "Emergency": Value Change {
                n250 = event-data() -> ()  [unwired: 1 in, 1 out]
                n251 = shared-variable "HX-CRIO-SECONDARY\\RTProjectLibrary.lvlib\\Emergency"("Emergency") -> ()  [unwired: 1 in, 1 out]
              }
              event "Force Idle": Value Change {
                n252 = event-data() -> ()  [unwired: 1 in, 1 out]
                n253 = shared-variable "HX-CRIO-SECONDARY\\RTProjectLibrary.lvlib\\ForceIdle"("Force Idle") -> ()  [unwired: 1 in, 1 out]
              }
              event "Vent Tanks": Value Change {
                n254 = event-data() -> ()  [unwired: 1 in, 1 out]
                n255 = shared-variable "HX-CRIO-SECONDARY\\RTProjectLibrary.lvlib\\VentTanks"("Vent Tanks") -> ()  [unwired: 1 in, 1 out]
              }
            }
            n256 = Tick Count (ms)() -> (millisecond timer value=w67:u32)
            n257 = local read "CurrentState"() -> (w64:T2)
            n258 = feedback #2(w67) -> (w70:u32)
            n259 = feedback-in #2(w67, FALSE) -> ()
            n260 = Subtract(x=w67, y=w70) -> (x-y=w69:u32)
            n261 = To Double Precision Float(number=w64) -> (double precision float=w63:dbl)
            n262 = global read "HostDataGLOBAL.vi" "Data"() -> (w71:dbl[])
            n263 = To Double Precision Float(number=w69) -> (double precision float=w68:dbl)
            n264 = Build Array (concatenate)(w68, w71, w63) -> (w65:dbl[])
          }
        }
        frame True {
        }
      }
    }
    frame #3 {
      w423 = T3."Enabled" ("Disabled")
      w405 = FALSE
      # "Resets all button controls\non the front panel after\ncompletion"
      n265 = local write "Abort"(w405) -> ()
      n266 = local write "Clear Error"(w405) -> ()
      n267 = local write "Idle to Ready"(w405) -> ()
      n268 = local write "Power On"(w405) -> ()
      n269 = local write "Stop Host"(w405) -> ()
      n270 = local write "Stop cRIO"(w405) -> ()
      n271 = local write "Emergency"(w405) -> ()
      n272 = local write "Vent Tanks"(w405) -> ()
      n273 = property on="Testing Mode?" class="Bool (strict)"("DisabledEnum"=w423) -> ()  [unwired: 2 in, 2 out]
      n274 = property on="Force Idle" class="Bool"("DisabledEnum"=w423) -> ()  [unwired: 2 in, 2 out]
      n275 = Get Date/Time In Seconds() -> (seconds since 1Jan1904=w420:timestamp)
      n276 = global read "HostDataGLOBAL.vi" "Labels"() -> (w404:string[])
      n277 = Format Date/Time String(time format string (%c)="%m%d %H%M%S", seconds (now)=w420) -> (date/time string=w409:string)  [unwired: 1 in]
      n278 = Build Array (concatenate)("Time (ms)" ("string"), w404) -> (w403:string[])
      n279 = Concatenate Strings("AquiredData\\data", w409) -> (w406:string)
      n280 = call <vilib>:"Application Directory.vi"() -> ("Application Directory"=w419:path)
      n281 = Concatenate Strings(w406, "(2).txt" ("string")) -> (w408:string)
      n282 = Concatenate Strings(w406, "(1).txt" ("string")) -> (w413:string)
      n283 = call <vilib>:"Application Directory.vi"() -> ("Application Directory"=w416:path)
      n284 = Build Array (concatenate)(w403, "Current State (Enum)" ("string")) -> (w401:string[])
      n285 = Build Path(base path=w419, name or relative path=w408) -> (appended path=w418:path)
      n286 = Build Path(base path=w416, name or relative path=w413) -> (appended path=w417:path)
      n287 = call-poly <vilib>:"Write Delimited Spreadsheet.vi"("file path (dialog if empty)"=w418, "1D data"=w401) -> ()  [unwired: 12 in, 2 out]
      n288 = call-poly <vilib>:"Write Delimited Spreadsheet.vi"("file path (dialog if empty)"=w417, "1D data"=w403) -> ()  [unwired: 12 in, 2 out]
      n289 = call-poly <vilib>:"Write Delimited Spreadsheet.vi"("file path (dialog if empty)"=w418, "2D data"=w412, "append to file? (new file:F)"=TRUE) -> ()  [unwired: 11 in, 2 out]
      n290 = call-poly <vilib>:"Write Delimited Spreadsheet.vi"("file path (dialog if empty)"=w417, "2D data"=w411, "append to file? (new file:F)"=TRUE) -> ()  [unwired: 11 in, 2 out]
    }
  }
